vi "Get FPGA Name from Script.vi"(1 "file":path, 4 "FPGA Interface":refnum<class "FPGA Interface.lvclass">) -> (0 "FPGA Name":string)   [LabVIEW 2026, in "TALOS.lvlib" / "Interfaces.lvlib" / "FPGA Interface.lvclass"]
uses:
  FPGA Interface.lvclass
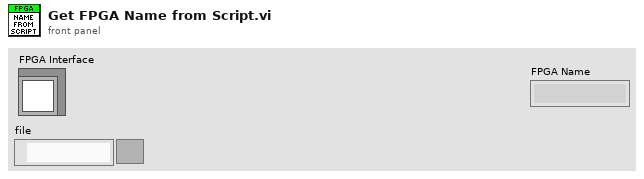
[diagram p1: front panel]
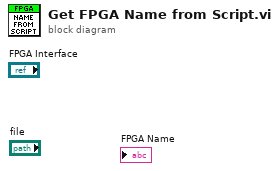
[diagram p0: block diagram]
diagram:
